vi "TerminationMonitorExample.vi"(11 "SequenceContext":refnum<k7>) -> (0 "Error Out":errorcluster)   [LabVIEW 2011]
doc: "This VI loops until either the Stop button is pressed or the calling TestStand sequence is terminated. The Termination Monitor VI allows this VI to query the TestStand execution for its current status."
panel:
  in  "Stop Button":bool
  # "This VI loops until either the Stop button is pressed or the calling TestStand sequence is terminated. The Termination Monitor VI allows this VI to query the TestStand execution for its current status."
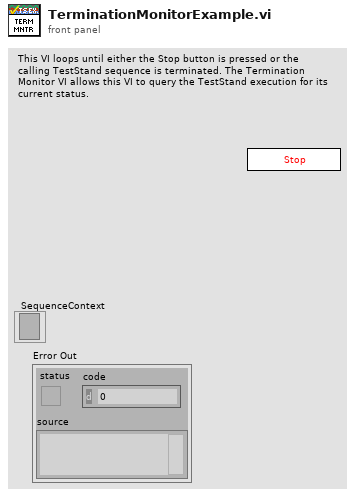
[diagram p1: front panel]
types:
  T1 = typedef "TestStand - Status Monitor.ctl" = cluster{"Sequence Context":refnum<k7>, "Execution":refnum<k7>, "Termination Monitor":refnum<k7>}
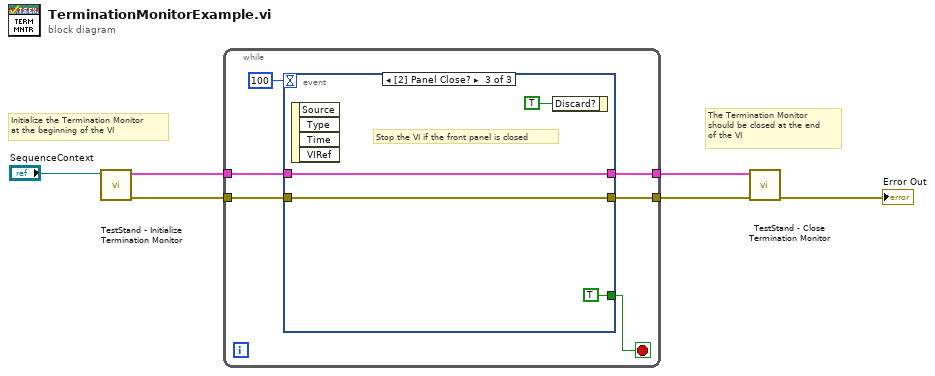
[diagram p0: block diagram]
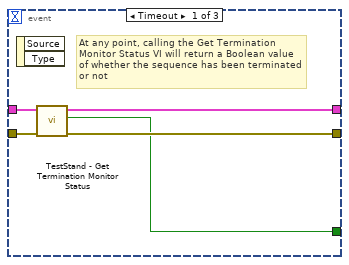
[diagram p2: hidden frame]
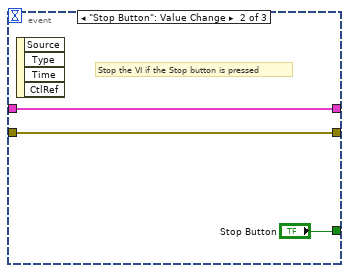
[diagram p3: hidden frame]
diagram:
  # "The Termination Monitor\nshould be closed at the end\nof the VI"
  # "Initialize the Termination Monitor\nat the beginning of the VI"
  n1 = call <vilib>:"TestStand - Initialize Termination Monitor.vi"("Sequence Context In"="SequenceContext") -> ("error out"=w4:errorcluster, "Status Monitor Out"=w5:T1)  [unwired: 9 in]
  n2 = while {
    tunnel: w5 -> [w11]
    tunnel: w4 -> [w10]
    tunnel: [w9] -> w3
    tunnel: [w8] -> w2
    stop <- w7 stop-if-true
    n3 = event shown="[2] Panel Close?" {
      selector: _ -> [_ _ _]
      dyn-events: _ -> [_ _ _]
      timeout: 100 -> [_ _ _]
      tunnel: w11 -> [w17 w19 w23]
      tunnel: w10 -> [w16 w18 w22]
      tunnel: [w15 w18 w22] -> w9
      tunnel: [w14 w19 w23] -> w8
      tunnel: [w13 "Stop Button" TRUE ("Stop Button")] -> w7
      event Timeout {
        # "At any point, calling the Get Termination\nMonitor Status VI will return a Boolean value\nof whether the sequence has been terminated \nor not"
        n4 = event-data() -> ()  [unwired: 1 in, 2 out]
        n5 = call <vilib>:"TestStand - Get Termination Monitor Status.vi"("error in (no error)"=w16, "Status Monitor In"=w17) -> ("error out"=w15:errorcluster, "Terminating or Aborting"=w13:bool, "Status Monitor Out"=w14:T1)  [unwired: 7 in]
      }
      event "Stop Button": Value Change {
        # "Stop the VI if the Stop button is pressed"
        n6 = event-data() -> ()  [unwired: 1 in, 4 out]
      }
      event Panel Close? {
        # "Stop the VI if the front panel is closed"
        n7 = event-data() -> ()  [unwired: 1 in, 4 out]
        n8 = event-data("Discard?"=TRUE) -> ()  [unwired: 1 in, 1 out]
      }
    }
  }
  n9 = call <vilib>:"TestStand - Close Termination Monitor.vi"("error in (no error)"=w3, "Status Monitor In"=w2) -> ("error out"=→"Error Out":errorcluster)  [unwired: 9 in]
